vi "Prog8.vi"() -> ()   [LabVIEW 2021]
panel:
  out "Array 2":string[](array[string])
  out "x = y? 2":bool
  out "x = y?":bool[](array[boolean])
  out "Array":string[](array[string])
  out "size(s)":i32
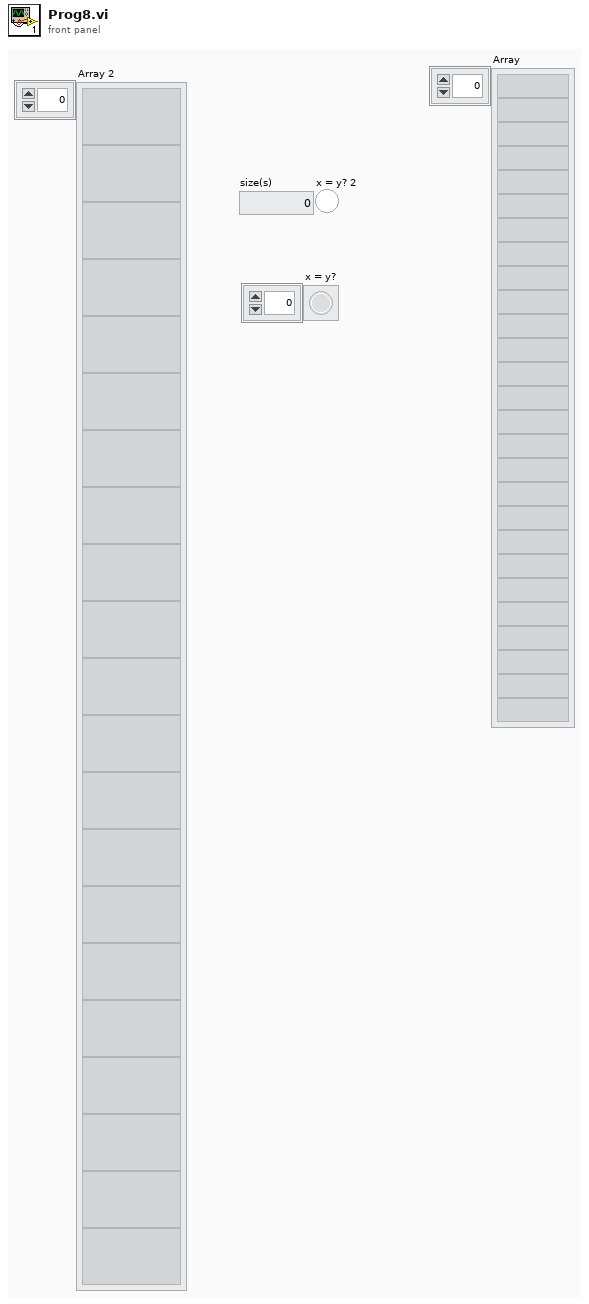
[diagram p1: front panel]
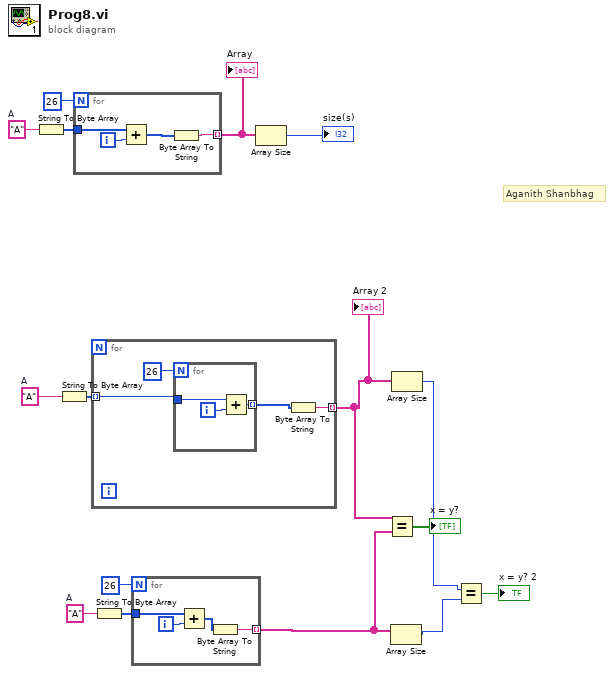
[diagram p0: block diagram]
diagram:
  w8 = "A"  # A
  w13 = "A"  # A
  w16 = "A"  # A
  # "Aganith Shanbhag"
  n1 = String To Byte Array(string=w16) -> (unsigned byte array=w15:u8[])
  n2 = String To Byte Array(string=w8) -> (unsigned byte array=w7:u8[])
  n3 = for {
    N: 26 -> [_]
    tunnel: w15 -> [w20]
    tunnel: [w17] -> w10 mode=indexing
    i -> [w19]
    n4 = Add(x=w20, y=w19) -> (x+y=w18:i32[])
    n5 = Byte Array To String(unsigned byte array=w18) -> (string=w17:string)
  }
  "Array" <- w10
  n6 = for {
    tunnel: w7 -> [w23] mode=indexing
    tunnel: [w21] -> w6 mode=indexing
    n7 = for {
      N: 26 -> [_]
      tunnel: w23 -> [w27]
      tunnel: [w25] -> w22 mode=indexing
      i -> [w26]
      n8 = Add(x=w27, y=w26) -> (x+y=w25:i32)
    }
    n9 = Byte Array To String(unsigned byte array=w22) -> (string=w21:string)
  }
  "Array 2" <- w6
  n10 = String To Byte Array(string=w13) -> (unsigned byte array=w12:u8[])
  n11 = for {
    N: 26 -> [_]
    tunnel: w12 -> [w31]
    tunnel: [w28] -> w5 mode=indexing
    i -> [w30]
    n12 = Add(x=w31, y=w30) -> (x+y=w29:i32[])
    n13 = Byte Array To String(unsigned byte array=w29) -> (string=w28:string)
  }
  n14 = Array Size(array=w10) -> (size(s)=→"size(s)":i32)
  n15 = Equal?(x=w6, y=w5) -> (x = y?=→"x = y?":bool[])
  n16 = Array Size(array=w5) -> (size(s)=w2:i32)
  n17 = Array Size(array=w6) -> (size(s)=w3:i32)
  n18 = Equal?(x=w3, y=w2) -> (x = y?=→"x = y? 2":bool)
